vi "Check Add Routing Channel Parameters.vi"(6 "Initial State":string="No Connections", 8 "error in (no error)":errorcluster, 9 "State Configurations":T1=[{"Name"="No Connections", "Description"="State with no connections", "Value"=-1, "Connection List"=[]}], 10 "Channel Name":string, 11 "Routing Channels Ref in":T4 format="%.0x") -> (0 "error out":errorcluster, 3 "Routing Channels Ref out":T4 format="%.0x")   [LabVIEW 2017, in "Routing and Faulting Scripting.lvlib"]
uses:
  Routing and Faulting Scripting.lvlib
  <vilib>/NI Veristand/Custom Device API/Custom Device Item Ref.ctl
  Shared/Channel States.ctl
  Shared/Routing State.ctl
  Shared/Connection.ctl
  <vilib>/NI VeriStand/Custom Device API/Custom Device API.lvlib
  Shared/Routing and Faulting Shared.lvlib
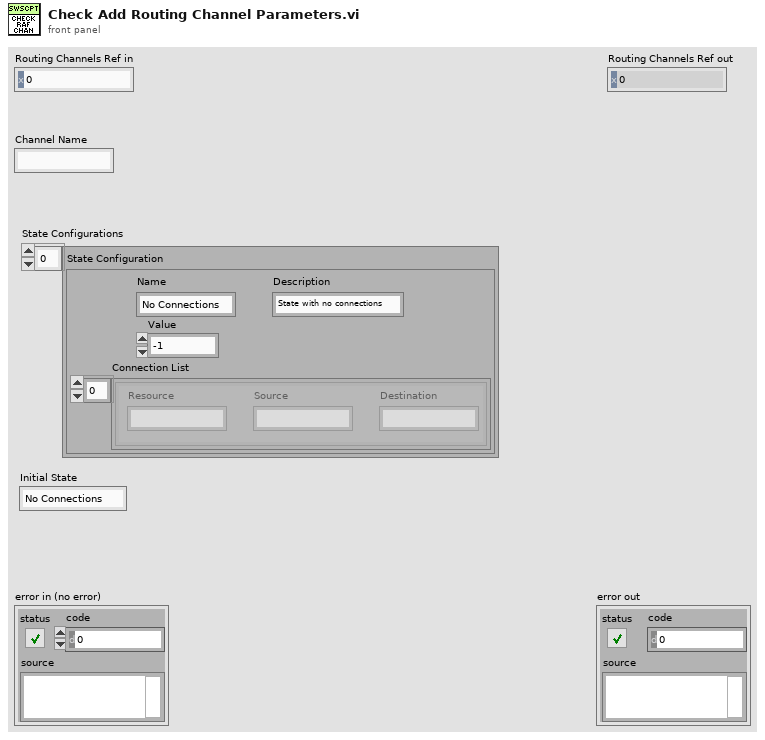
[diagram p1: front panel]
types:
  T1 = typedef "Routing and Faulting Shared.lvlib/Channel States.ctl" = T2[]
  T2 = typedef "Routing and Faulting Shared.lvlib/Routing State.ctl" = cluster{"Name":string, "Description":string, "Value":i32, "Connection List":T3[]}
  T3 = typedef "Routing and Faulting Shared.lvlib/Connection.ctl" = cluster{"Resource":string, "Source":string, "Destination":string}
  T4 = typedef "Custom Device API.lvlib/Custom Device Item Ref.ctl" = u64
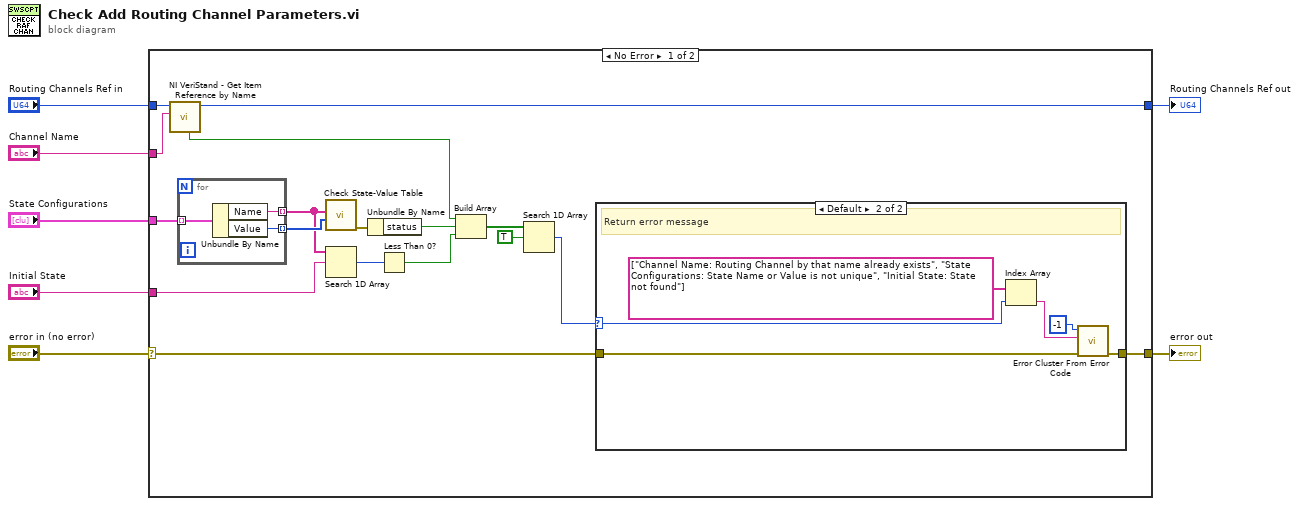
[diagram p0: block diagram]
diagram:
  n1 = case shown="No Error" "error in (no error)" {
    selector: "error in (no error)" -> [w10 w36]
    tunnel: [w9 w36] -> w7
    tunnel: "Routing Channels Ref in" -> [w19 w35]
    tunnel: "Channel Name" -> [w18 _]
    tunnel: "State Configurations" -> [w24 _]
    tunnel: "Initial State" -> [w21 _]
    tunnel: [w8 w35] -> w1
    frame No Error {
      n2 = call <vilib>:"NI VeriStand - Get Item Reference by Name.vi"("Item Name"=w18, "Parent Ref in"=w19) -> ("Parent Ref out"=w8:T4, "Found"=w16:bool)  [unwired: 6 in, 2 out]
      n3 = for {
        tunnel: w24 -> [w34] mode=indexing
        tunnel: [w33] -> w22 mode=indexing
        tunnel: [w32] -> w23 mode=indexing
        n4 = Unbundle By Name(w34) -> ("Name"=w33:string, "Value"=w32:i32)
      }
      n5 = call "Check State-Value Table.vi"("State Values"=w23, "State Names"=w22) -> ("error out"=w15:errorcluster)  [unwired: 8 in, 1 out]
      n6 = Search 1D Array(1D array=w22, element=w21) -> (index of element=w20:i32)  [unwired: 1 in]
      n7 = Unbundle By Name(w15) -> ("status"=w14:bool)
      n8 = Less Than 0?(x=w20) -> (x < 0?=w13:bool)
      n9 = Build Array(w16, w14, w13) -> (w12:bool[])
      n10 = Search 1D Array(1D array=w12, element=TRUE) -> (index of element=w11:i32)  [unwired: 1 in]
      n11 = case shown="Default" w11 {
        selector: w11 -> [_ w28]
        tunnel: w10 -> [w25 w30]
        tunnel: [w25 w26] -> w9
        frame -1 {
          # "All checks pass - No Error"
        }
        frame Default {
          # "Return error message"
          n12 = Index Array(array=string[] ["Channel Name: Routing Channel by that name already exists", "State Configurations: State Name or Value is not unique", "Initial State: State not found"], index=w28) -> (element=w27:string)
          n13 = call <vilib>:"Error Cluster From Error Code.vi"("error in (no error)"=w30, "error message (\"\")"=w27, "error code (0)"=-1) -> ("error out"=w26:errorcluster)  [unwired: 6 in]
        }
      }
    }
    frame Error {
    }
  }
  "error out" <- w7
  "Routing Channels Ref out" <- w1
